vi "WriteFile.vi"(1 "Detector Select":enum32{"4 Detectors", "8 Detectors"}(radio)=enum."8 Detectors", 2 "Intensity data":string, 3 "Tau data":string, 4 "g2 data":string, 6 "Scan":u32, 7 "X Index":u32, 8 "Data Save Directory:":path=path "C:/Data/test", 9 "Y Index":u32, 10 "File Name:":string="tst8", 11 "Optical Input":u32, 13 "Optical Output":u32) -> (14 "Computer Time":string="2009-8-25 9:52:59", 19 "error out":errorcluster)   [LabVIEW 2011]
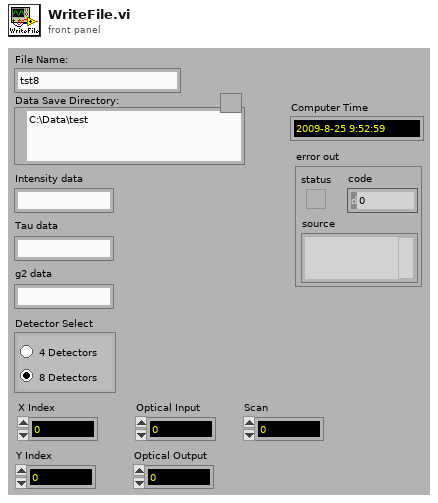
[diagram p1: front panel]
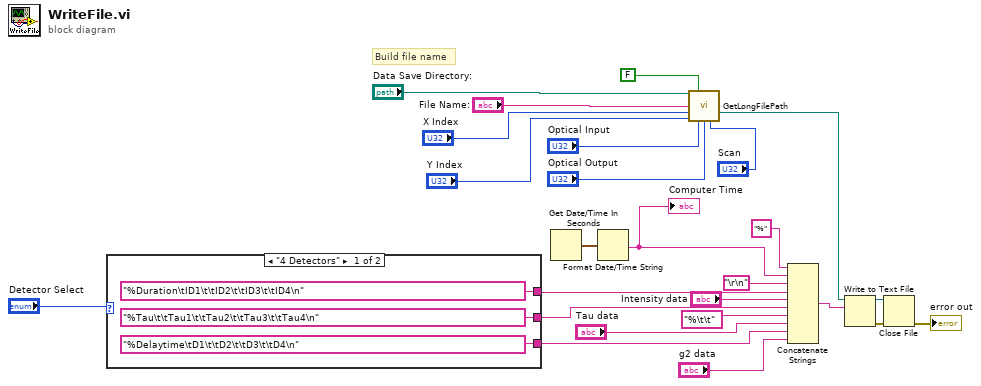
[diagram p0: block diagram]
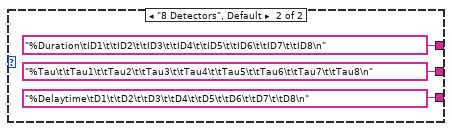
[diagram p2: hidden frame]
diagram:
  # "Build file name"
  n1 = case shown="\"4 Detectors\"" "Detector Select" {
    tunnel: ["%Duration\tID1\t\tID2\t\tID3\t\tID4\n" "%Duration\tID1\t\tID2\t\tID3\t\tID4\t\tID5\t\tID6\t\tID7\t\tID8\n"] -> w21
    tunnel: ["%Tau\t\tTau1\t\tTau2\t\tTau3\t\tTau4\n" "%Tau\t\tTau1\t\tTau2\t\tTau3\t\tTau4\t\tTau5\t\tTau6\t\tTau7\t\tTau8\n"] -> w20
    tunnel: ["%Delaytime\tD1\t\tD2\t\tD3\t\tD4\n" "%Delaytime\tD1\t\tD2\t\tD3\t\tD4\t\tD5\t\tD6\t\tD7\t\tD8\n"] -> w12
    frame "4 Detectors" {
    }
    frame "8 Detectors", Default {
    }
  }
  n2 = Get Date/Time In Seconds() -> (seconds since 1Jan1904=w25:timestamp)
  n3 = Format Date/Time String(seconds (now)=w25) -> (date/time string=w13:string)  [unwired: 2 in]
  "Computer Time" <- w13
  n4 = call "GetLongFilePath.vi"("path"="Data Save Directory:", "replace \\ by \\\\"=FALSE, "file name"="File Name:", "X Row"="X Index", "Y Row"="Y Index", "Optical Input"="Optical Input", "Optical Output"="Optical Output", "Scan"="Scan") -> ("complete path"=w8:path)  [unwired: 6 in, 1 out]
  n5 = Concatenate Strings("%", w13, "\r\n", w21, "Intensity data", w20, "%\t\t", "Tau data", w12, "g2 data") -> (w22:string)
  n6 = Write to Text File(file (use dialog)=w8, text=w22) -> (refnum out=w18:refnum<file>, error out=w19:errorcluster)  [unwired: 2 in, 1 out]
  n7 = Close File(refnum=w18, error in=w19) -> (error out=→"error out":errorcluster)  [unwired: 1 out]
